vi "AO(Read).vi"() -> ()   [LabVIEW 2023]
uses:
  <instrlib>/HandsOnPi2040/Public/PWMSettings.ctl
  <instrlib>/HandsOnPi2040/Public/AOs.ctl
  <instrlib>/HandsOnPi2040/HandsOnPi2040.lvlib
panel:
  in  "stop":bool
  out "AnOutValues":T1
  in  "Duty":sgl(slide) scale=0.0..1.0
  in  "Frequency":sgl(slide) scale=10.0..500000.0
  out "error out":errorcluster
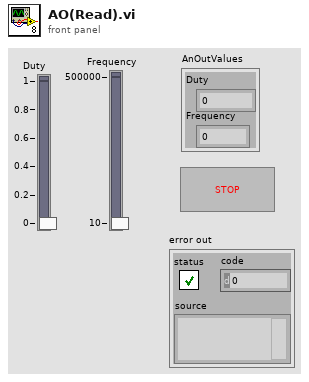
[diagram p1: front panel]
types:
  T1 = typedef "HandsOnPi2040.lvlib/PWMSettings.ctl" = cluster{"Duty":sgl, "Frequency":sgl}
  T2 = typedef "HandsOnPi2040.lvlib/AOs.ctl" = enum16{"No AO - Error", "AO1 (GPIO28)"}
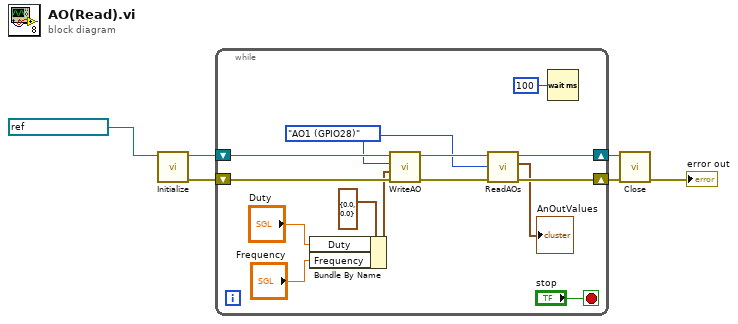
[diagram p0: block diagram]
diagram:
  n1 = call <instrlib>:"Initialize.vi"("VISA resource name"=refnum<visa-resource-name> "ASRL5::INSTR") -> ("error out"=w3:errorcluster, "VISA resource name out"=w4:refnum<visa-resource-name>)  [unwired: 8 in, 1 out]
  n2 = while {
    shift-right: [w12] -> w5
    shift-left: w4 -> [w20]
    shift-right: [w13] -> w6
    shift-left: w3 -> [w19]
    stop <- "stop" stop-if-true
    w8 = AOs."AO1 (GPIO28)" ("Analog Output")
    n3 = Bundle By Name(cluster=T1 {"Duty"=0.0, "Frequency"=0.0} ("PWM Settings"), "Duty"="Duty", "Frequency"="Frequency") -> (w17:T1)
    n4 = call <instrlib>:"WriteAO.vi"("error in (no error)"=w19, "PWM Settings"=w17, "Analog Output"=w8, "VISA resource name"=w20) -> ("error out"=w10:errorcluster, "VISA resource name out"=w11:refnum<visa-resource-name>)  [unwired: 6 in]
    n5 = call <instrlib>:"ReadAOs.vi"("error in (no error)"=w10, "Analog Output"=w8, "VISA resource name"=w11) -> ("error out"=w13:errorcluster, "AnOutValues"=→"AnOutValues":T1, "VISA resource name out"=w12:refnum<visa-resource-name>)  [unwired: 6 in]
    n6 = Wait (ms)(milliseconds to wait=u32 100) -> ()  [unwired: 1 out]
  }
  n7 = call <instrlib>:"Close.vi"("error in (no error)"=w6, "VISA resource name"=w5) -> ("error out"=→"error out":errorcluster)  [unwired: 9 in]
